vi "2 Ball Side Half.vi"(1 "Run?":bool) -> (0 "Done?":bool)   [LabVIEW 2013]
uses:
  Globals/Homes.vi
  Globals/Useful Values.vi
panel:
  out "Time Elapsed":dbl
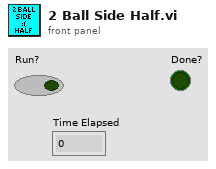
[diagram p1: front panel]
types:
  T1 = typedef "WPI_I2CDevRef.ctl" = cluster{"DevStatus":errorcluster, "Digital Module":T2, "Device Address":u8}
  T2 = typedef "FPGA_TypedefDigitalModule.ctl" = enum16{"Digital Module 1", "Digital Module 2"}
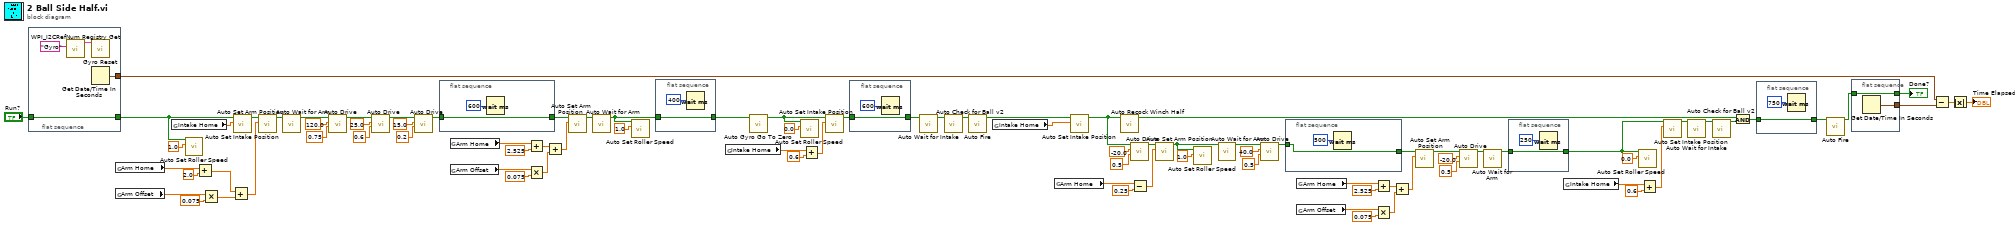
[diagram p0: block diagram]
diagram:
  n1 = flat-sequence {
    tunnel: "Run?" -> [w93]
    tunnel: [w93] -> w30
    tunnel: [w92] -> w54
    frame #0 {
      n2 = call <vilib>:"WPI_I2CRefNum Registry Get.vi"("refnum name"="Gyro") -> ("I2CDevRef"=w90:T1)  [unwired: 9 in, 1 out]
      n3 = call "Gyro Reset.vi"("I2CDevRef"=w90) -> ()  [unwired: 10 in, 1 out]
      n4 = Get Date/Time In Seconds() -> (seconds since 1Jan1904=w92:timestamp)
    }
  }
  n5 = global read "Homes.vi" "Arm Home"() -> (w88:dbl)
  n6 = global read "Useful Values.vi" "Arm Offset"() -> (w84:dbl)
  n7 = global read "Homes.vi" "Intake Home"() -> (w87:dbl)
  n8 = call "Auto Set Roller Speed.vi"("Value"=1.0, "Run?"=w30) -> ()  [unwired: 9 in, 1 out]
  n9 = Add(x=w88, y=2.0) -> (x+y=w83:dbl)
  n10 = Multiply(x=w84, y=0.075) -> (x*y=w86:dbl)
  n11 = Add(x=w83, y=w86) -> (x+y=w21:dbl)
  n12 = call "Auto Set Intake Position.vi"("Intake Position"=w87, "Run?"=w30) -> ("Done"=w20:bool)  [unwired: 9 in]
  n13 = call "Auto Set Arm Position.vi"("Arm Position"=w21, "Run?"=w20) -> ("Done"=w2:bool)  [unwired: 9 in]
  n14 = call "Auto Wait for Arm.vi"("Run?"=w2) -> ("Done"=w1:bool)  [unwired: 10 in]
  n15 = call "Auto Drive.vi"("Speed"=0.75, "Amount"=120.0, "Run?"=w1) -> ("Done"=w23:bool)  [unwired: 8 in]
  n16 = call "Auto Drive.vi"("Speed"=0.6, "Amount"=25.0, "Run?"=w23) -> ("Done"=w22:bool)  [unwired: 8 in]
  n17 = call "Auto Drive.vi"("Speed"=0.2, "Amount"=15.0, "Run?"=w22) -> ("Done"=w35:bool)  [unwired: 8 in]
  n18 = flat-sequence {
    tunnel: w35 -> [w94]
    tunnel: [w94] -> w70
    frame #0 {
      n19 = Wait (ms)(milliseconds to wait=u32 600) -> ()  [unwired: 1 out]
    }
  }
  n20 = global read "Homes.vi" "Arm Home"() -> (w74:dbl)
  n21 = global read "Useful Values.vi" "Arm Offset"() -> (w79:dbl)
  n22 = Add(x=w74, y=2.525) -> (x+y=w80:dbl)
  n23 = Multiply(x=w79, y=0.075) -> (x*y=w77:dbl)
  n24 = Add(x=w80, y=w77) -> (x+y=w75:dbl)
  n25 = call "Auto Set Arm Position.vi"("Arm Position"=w75, "Run?"=w70) -> ("Done"=w73:bool)  [unwired: 9 in]
  n26 = call "Auto Wait for Arm.vi"("Run?"=w73) -> ("Done"=w18:bool)  [unwired: 10 in]
  n27 = call "Auto Set Roller Speed.vi"("Value"=1.0, "Run?"=w18) -> ()  [unwired: 9 in, 1 out]
  n28 = flat-sequence {
    tunnel: [w96] -> w4
    tunnel: w18 -> [w96]
    frame #0 {
      n29 = Wait (ms)(milliseconds to wait=u32 400) -> ()  [unwired: 1 out]
    }
  }
  n30 = global read "Homes.vi" "Intake Home"() -> (w51:dbl)
  n31 = call "Auto Gyro Go To Zero.vi"("Run?"=w4) -> ("Done"=w3:bool)  [unwired: 10 in]
  n32 = call "Auto Set Roller Speed.vi"("Value"=0.0, "Run?"=w3) -> ()  [unwired: 9 in, 1 out]
  n33 = Add(x=w51, y=0.6) -> (x+y=w49:dbl)
  n34 = call "Auto Set Intake Position.vi"("Intake Position"=w49, "Run?"=w3) -> ("Done"=w37:bool)  [unwired: 9 in]
  n35 = flat-sequence {
    tunnel: [w98] -> w38
    tunnel: w37 -> [w98]
    frame #0 {
      n36 = Wait (ms)(milliseconds to wait=u32 600) -> ()  [unwired: 1 out]
    }
  }
  n37 = call "Auto Wait for Intake.vi"("Run?"=w38) -> ("Done"=w44:bool)  [unwired: 10 in]
  n38 = call "Auto Check for Ball v2.vi"("Run?"=w44) -> ("Done"=w69:bool)  [unwired: 10 in]
  n39 = call "Auto Fire.vi"("Run?"=w69) -> ("Done"=w42:bool)  [unwired: 10 in]
  n40 = global read "Homes.vi" "Intake Home"() -> (w41:dbl)
  n41 = global read "Homes.vi" "Arm Home"() -> (w68:dbl)
  n42 = call "Auto Set Intake Position.vi"("Intake Position"=w41, "Run?"=w42) -> ("Done"=w15:bool)  [unwired: 9 in]
  n43 = call "Auto Recock Winch Half.vi"("Run?"=w15) -> ("Done"=w57:bool)  [unwired: 10 in]
  n44 = call "Auto Drive.vi"("Speed"=0.5, "Amount"=-20.0, "Run?"=w15) -> ("Done"=w14:bool)  [unwired: 8 in]
  n45 = Subtract(x=w68, y=0.25) -> (x-y=w66:dbl)
  n46 = call "Auto Set Arm Position.vi"("Arm Position"=w66, "Run?"=w14) -> ("Done"=w31:bool)  [unwired: 9 in]
  n47 = call "Auto Set Roller Speed.vi"("Value"=1.0, "Run?"=w31) -> ()  [unwired: 9 in, 1 out]
  n48 = call "Auto Wait for Arm.vi"("Run?"=w31) -> ("Done"=w11:bool)  [unwired: 10 in]
  n49 = call "Auto Drive.vi"("Speed"=0.5, "Amount"=40.0, "Run?"=w11) -> ("Done"=w10:bool)  [unwired: 8 in]
  n50 = flat-sequence {
    tunnel: w10 -> [w100]
    tunnel: [w100] -> w9
    frame #0 {
      n51 = Wait (ms)(milliseconds to wait=u32 500) -> ()  [unwired: 1 out]
    }
  }
  n52 = global read "Homes.vi" "Arm Home"() -> (w65:dbl)
  n53 = global read "Useful Values.vi" "Arm Offset"() -> (w61:dbl)
  n54 = Add(x=w65, y=2.525) -> (x+y=w60:dbl)
  n55 = Multiply(x=w61, y=0.075) -> (x*y=w63:dbl)
  n56 = Add(x=w60, y=w63) -> (x+y=w59:dbl)
  n57 = call "Auto Set Arm Position.vi"("Arm Position"=w59, "Run?"=w9) -> ("Done"=w6:bool)  [unwired: 9 in]
  n58 = call "Auto Drive.vi"("Speed"=0.5, "Amount"=-20.0, "Run?"=w6) -> ("Done"=w5:bool)  [unwired: 8 in]
  n59 = call "Auto Wait for Arm.vi"("Run?"=w5) -> ("Done"=w27:bool)  [unwired: 10 in]
  n60 = flat-sequence {
    tunnel: w27 -> [w102]
    tunnel: [w102] -> w26
    frame #0 {
      n61 = Wait (ms)(milliseconds to wait=u32 250) -> ()  [unwired: 1 out]
    }
  }
  n62 = global read "Homes.vi" "Intake Home"() -> (w45:dbl)
  n63 = call "Auto Set Roller Speed.vi"("Value"=0.0, "Run?"=w26) -> ()  [unwired: 9 in, 1 out]
  n64 = Add(x=w45, y=0.6) -> (x+y=w47:dbl)
  n65 = call "Auto Set Intake Position.vi"("Intake Position"=w47, "Run?"=w26) -> ("Done"=w48:bool)  [unwired: 9 in]
  n66 = call "Auto Wait for Intake.vi"("Run?"=w48) -> ("Done"=w43:bool)  [unwired: 10 in]
  n67 = call "Auto Check for Ball v2.vi"("Run?"=w43) -> ("Done"=w58:bool)  [unwired: 10 in]
  n68 = And(x=w57, y=w58) -> (x .and. y?=w29:bool)
  n69 = flat-sequence {
    tunnel: w29 -> [w104]
    tunnel: [w104] -> w28
    frame #0 {
      n70 = Wait (ms)(milliseconds to wait=u32 750) -> ()  [unwired: 1 out]
    }
  }
  n71 = call "Auto Fire.vi"("Run?"=w28) -> ("Done"=w32:bool)  [unwired: 10 in]
  n72 = flat-sequence {
    tunnel: w32 -> [w107]
    tunnel: [w107] -> w56
    tunnel: [w106] -> w55
    frame #0 {
      n73 = Get Date/Time In Seconds() -> (seconds since 1Jan1904=w106:timestamp)
    }
  }
  n74 = Subtract(x=w54, y=w55) -> (x-y=w53:dbl)
  n75 = Absolute Value(x=w53) -> (abs(x)=→"Time Elapsed":dbl)
  "Done?" <- w56
